vi "BioMapWriteCore.vi"(6 "conv. coeff.":sgl=655.0, 7 "Image in":dbl[][][](array[numeric]), 8 "error in":errorcluster, 9 "Y_img":i32, 10 "Image Params":T1={"File Header"={"Start Position"=[], "StepWidth"=[0.05, 0.05], "Dimension"=[], "SpecLength"=10000}, "mzCali."=[0.0, 1.0, 0.0], "m/z_Array"=[0.0, 1.0, 0.0], "SampleRate"=0.0, "TrigDelay"=0.0, "file refnum"=refnum, "file path"=path "", "PeakOI"=[], "Binning"={"Enable"=FALSE, "BinType"=enum."ByScreen", "BinWidth"=0.5, "Maximum"=0.0, "Minimum"=0.0}} {"SampleRate" items=["50MS/s"=50000000.0, "100MS/s"=100000000.0, "125MS/s"=125000000.0, "200MS/s"=200000000.0, "250MS/s"=250000000.0, "500MS/s"=500000000.0, "1GS/s"=1000000000.0, "1.6GS/s"=1600000000.0, "2GS/s"=2000000000.0, "4GS/s"=4000000000.0]}, 11 "data buffer in":refnum<queue>) -> (0 "error out":errorcluster, 2 "file refnum out":refnum<file>, 5 "Image out":dbl[][][](array[numeric]))   [LabVIEW 2014]
uses:
  BioMAPWriterCoreParams.ctl
  Files/BinaryHeader.ctl
  ControlDef/SampleRateSelector.ctl
  Binning/BinType.ctl
panel:
  out "#element":i32
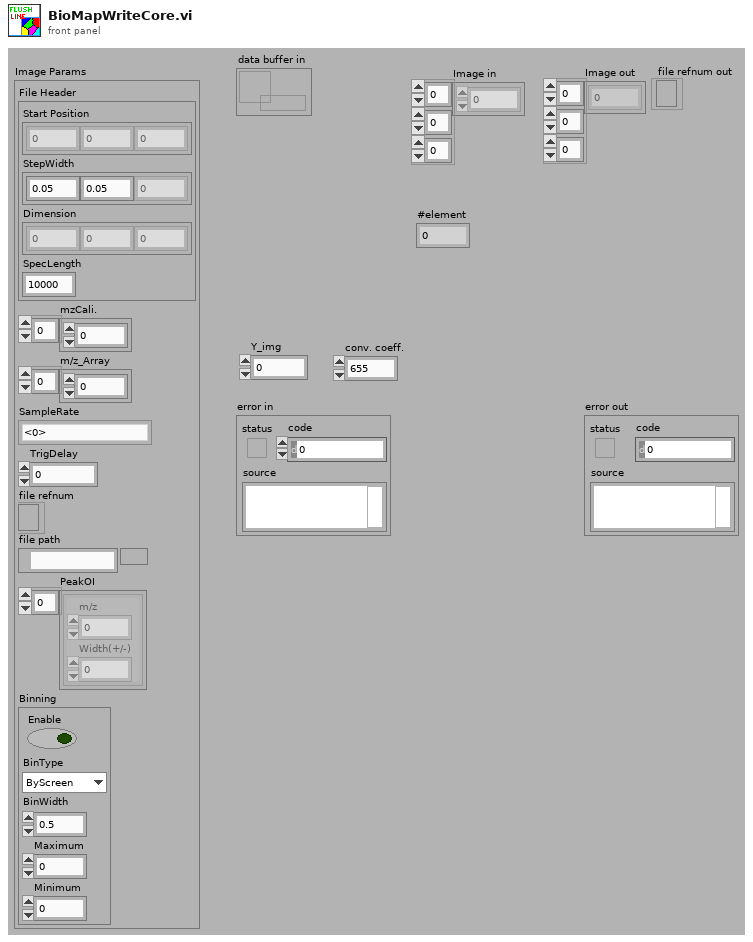
[diagram p1: front panel]
types:
  T1 = typedef "BioMAPWriterCoreParams.ctl" = cluster{"File Header":T2, "mzCali.":dbl[], "m/z_Array":dbl[], "SampleRate":T3, "TrigDelay":dbl, "file refnum":refnum<file>, "file path":path, "PeakOI":cluster{"m/z":dbl, "Width(+/-)":dbl}[], "Binning":cluster{"Enable":bool, "BinType":T4, "BinWidth":dbl, "Maximum":dbl, "Minimum":dbl}}
  T2 = typedef "BinaryHeader.ctl" = cluster{"Start Position":dbl[], "StepWidth":dbl[], "Dimension":i32[], "SpecLength":i32}
  T3 = typedef "SampleRateSelector.ctl" = dbl
  T4 = typedef "BinType.ctl" = enum16{"ByTime", "ByScreen", "ByMass", "ToUnitMass"}
  T5 = enum16{"big-endian, network order", "native, host order", "little-endian"}
  T6 = cluster{"Average":i32, "X (Img)":i32, "Y (Img)":i32, "Spectra":sgl[]}[]
  T7 = cluster{"Average":i32, "X (Img)":i32, "Y (Img)":i32, "Spectra":sgl[]}
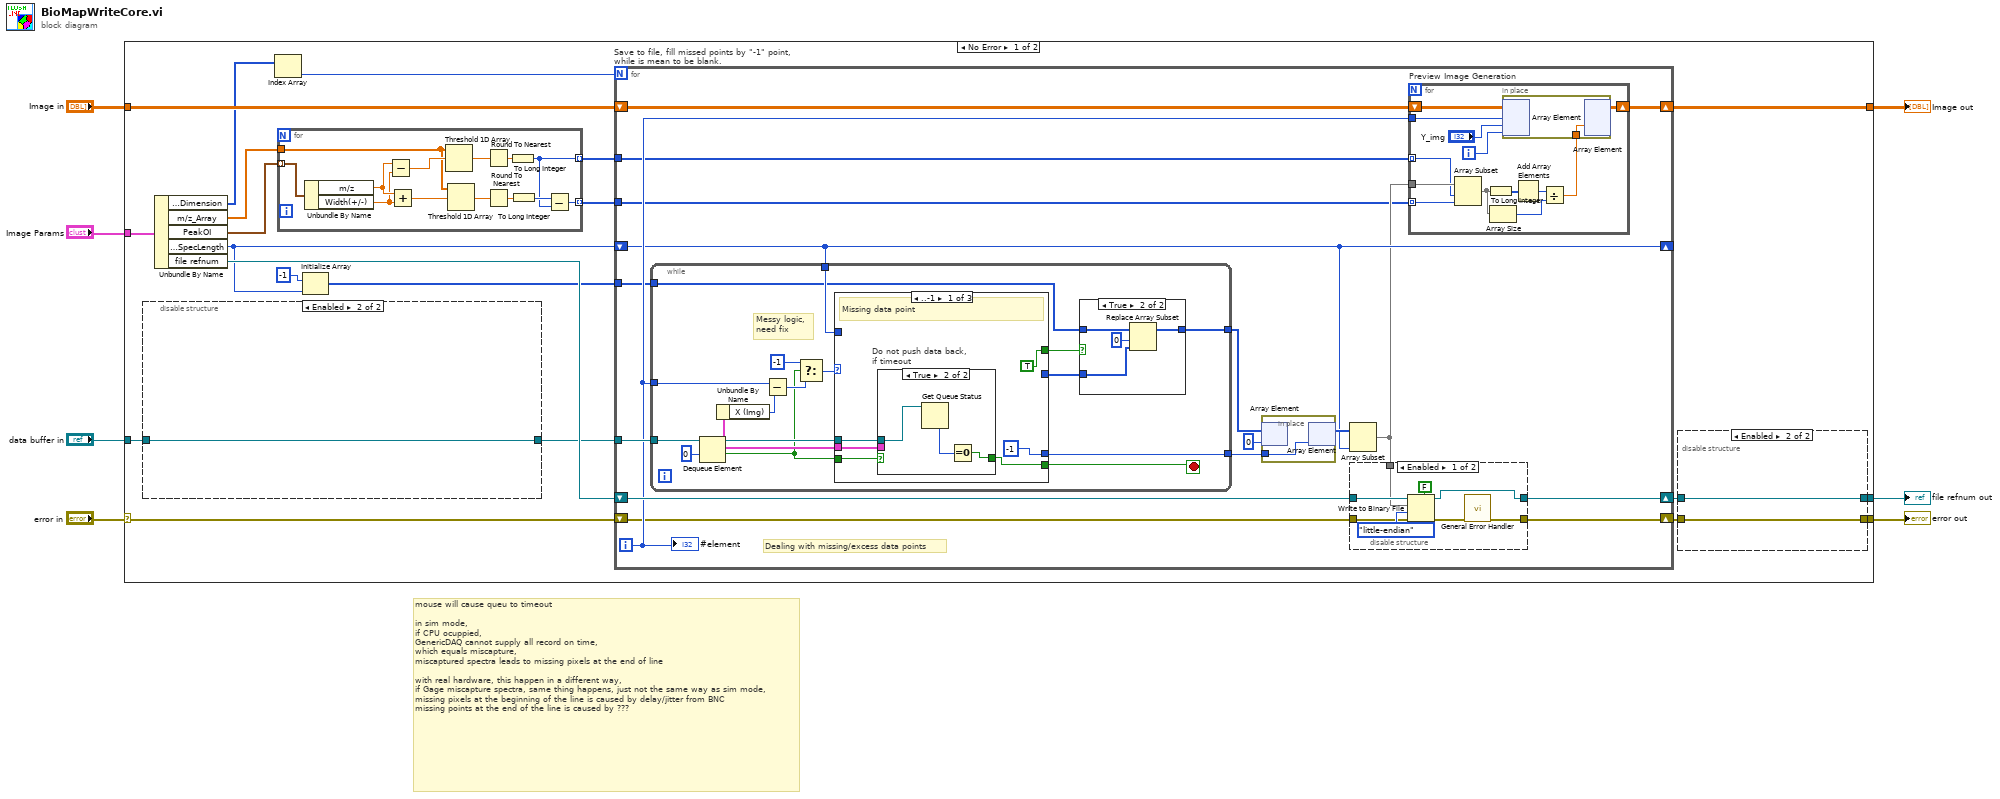
[diagram p0: block diagram]
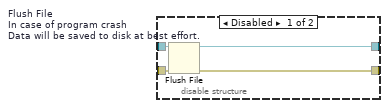
[diagram p2: hidden frame]
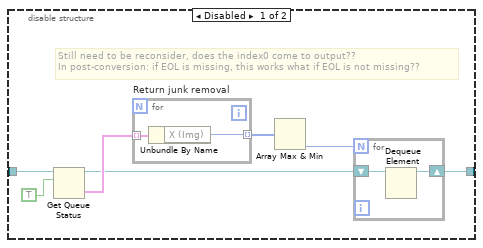
[diagram p3: hidden frame]
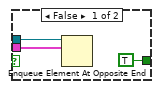
[diagram p6: hidden frame]
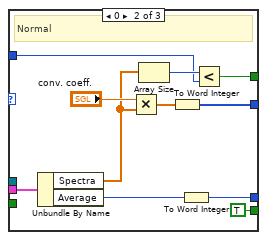
[diagram p7: hidden frame]
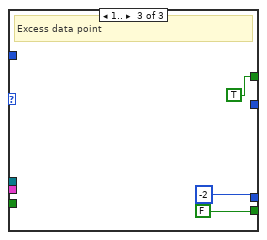
[diagram p8: hidden frame]
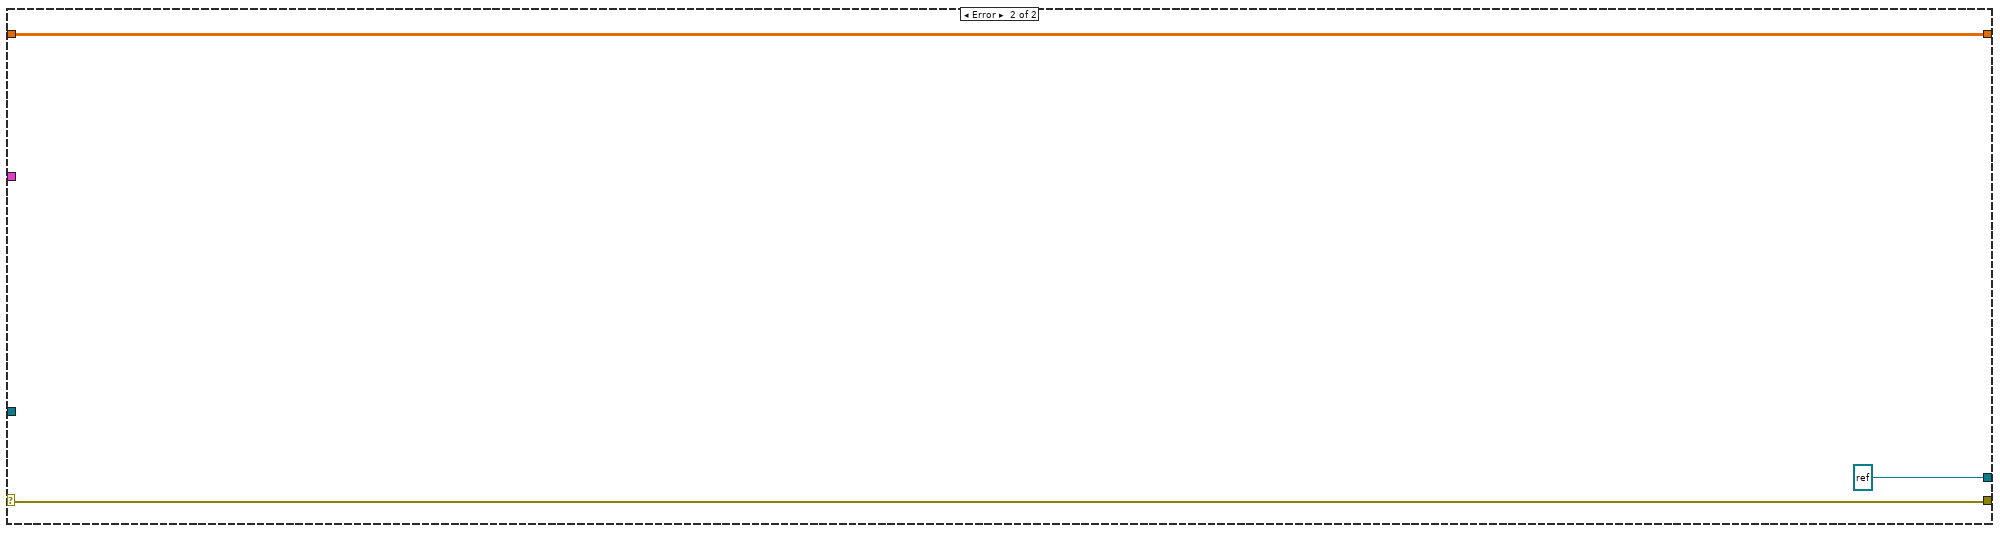
[diagram p9: hidden frame]
diagram:
  # "mouse will cause queu to timeout\n\nin sim mode, \nif CPU ocuppied,\nGenericDAQ cannot supply all record on time,\nwhich equals miscapture,\nmiscaptured spectra leads to missing pixels at the end of line\n\nwith real hardware, this happen in a different way,\nif Gage miscapture spectra, same thing happens, just not the same way as sim mode,\nmissing pixels at the beginning of the line is caused by delay/jitter from BNC\nmissing points at the end of the line is caused by ???"
  n1 = case shown="No Error" "error in" {
    selector: "error in" -> [w24 w150]
    tunnel: [w27 w148] -> w7
    tunnel: [w15 w150] -> w6
    tunnel: [w17 refnum<file> refnum ("file refnum")] -> w5
    tunnel: "Image in" -> [w25 w148]
    tunnel: "data buffer in" -> [w14 _]
    tunnel: "Image Params" -> [w12 _]
    frame No Error {
      n2 = disable-structure shown="Enabled" {
        disable-tunnel: w14 -> [w51 w58]
        disable-tunnel: [w49 w58] -> w20
        frame Disabled {
          # "Still need to be reconsider, does the index0 come to output??\nIn post-conversion: if EOL is missing, this works what if EOL is not missing??"
          # "Dealing with uncontroled laser. Data points from stage returning will be ignored."
          n3 = Get Queue Status(queue=w51, return elements? (F)=TRUE) -> (queue out=w50:refnum<queue>, elements=w53:T6)  [unwired: 1 in, 6 out]
          n4 = for "Return junk removal" {
            tunnel: w53 -> [w57] mode=indexing
            tunnel: [w56] -> w48 mode=indexing
            n5 = Unbundle By Name(w57) -> ("X (Img)"=w56:i32)
          }
          n6 = Array Max & Min(array=w48) -> (min index (indices)=w47:i32)  [unwired: 3 out]
          n7 = for {
            N: w47 -> [_]
            shift-right: [w54] -> w49
            shift-left: w50 -> [w55]
            n8 = Dequeue Element(queue=w55) -> (queue out=w54:refnum<queue>)  [unwired: 2 in, 3 out]
          }
        }
        frame Enabled {
          # "batch binning"
        }
      }
      n9 = Unbundle By Name(w12) -> ("File Header.Dimension"=w23:i32[], "m/z_Array"=w11:dbl[], "PeakOI"=w10:cluster{"m/z":dbl, "Width(+/-)":dbl}[], "File Header.SpecLength"=w13:i32, "file refnum"=w22:refnum<file>)
      n10 = Index Array(array=w23) -> (element=w21:i32)  [unwired: 1 in]
      n11 = for "Preview Image Generation" {
        tunnel: w10 -> [w46] mode=indexing
        tunnel: w11 -> [w42]
        tunnel: [w35] -> w9 mode=indexing
        tunnel: [w34] -> w8 mode=indexing
        n12 = Unbundle By Name(w46) -> ("m/z"=w45:dbl, "Width(+/-)"=w44:dbl)
        n13 = Subtract(x=w45, y=w44) -> (x-y=w43:dbl)
        n14 = Add(x=w45, y=w44) -> (x+y=w41:dbl)
        n15 = Threshold 1D Array(2:w43, 3:w42) -> (0:w40:dbl)  [unwired: 1 in]
        n16 = Threshold 1D Array(2:w41, 3:w42) -> (0:w39:dbl)  [unwired: 1 in]
        n17 = Round To Nearest(number=w40) -> (nearest integer value=w37:dbl)
        n18 = Round To Nearest(number=w39) -> (nearest integer value=w38:dbl)
        n19 = To Long Integer(number=w37) -> (32bit integer=w35:i32)
        n20 = To Long Integer(number=w38) -> (32bit integer=w36:i32)
        n21 = Subtract(x=w36, y=w35) -> (x-y=w34:i32)
      }
      n22 = Initialize Array(i16 -1 ("element"), w13) -> (w18:i16[])
      n23 = for "Save to file, fill missed points by \"-1\" point, while is mean to be blank." {
        N: w21 -> [_]
        shift-right: [w70] -> w16
        shift-left: w24 -> [w63]
        shift-right: [w72] -> w27
        shift-left: w25 -> [w71]
        tunnel: w20 -> [w75]
        shift-right: [w73] -> w26
        shift-left: w22 -> [w74]
        tunnel: w8 -> [w59]
        tunnel: w9 -> [w60]
        tunnel: w18 -> [w64]
        shift-right: [w62] -> _
        shift-left: w13 -> [w62]
        i -> [w65]
        # "Dealing with missing/excess data points"
        n24 = while {
          tunnel: w75 -> [w101]
          tunnel: [w95] -> w67
          tunnel: w62 -> [w94]
          tunnel: [w89] -> w66
          tunnel: w65 -> [w90]
          tunnel: w64 -> [w87]
          stop <- w93 stop-if-true
          # "Messy logic,\nneed fix"
          n25 = Dequeue Element(queue=w101, timeout in ms (-1)=0) -> (queue out=w97:refnum<queue>, element=w96:T7, timed out?=w86:bool)  [unwired: 1 in, 1 out]
          n26 = Unbundle By Name(w96) -> ("X (Img)"=w99:i32)
          n27 = Subtract(x=w90, y=w99) -> (x-y=w98:i32)
          n28 = Select(t=-1, s=w86, f=w98) -> (s? t:f=w92:i32)
          n29 = case shown="..-1" w92 {
            tunnel: w97 -> [w110 _ _]
            tunnel: w96 -> [w109 w129 _]
            tunnel: [i16 -1 ("Average") w127 i16 -2 ("Average")] -> w95
            tunnel: w94 -> [_ w122 _]
            tunnel: [w107 TRUE FALSE] -> w93
            tunnel: [_ w121 _] -> w88
            tunnel: [TRUE w120 TRUE] -> w85
            tunnel: w86 -> [w108 _ _]
            frame ..-1 {
              # "Missing data point"
              n30 = case "Do not push data back, \nif timeout" shown="True" w108 {
                tunnel: w110 -> [w115 w118]
                tunnel: w109 -> [w114 _]
                tunnel: [TRUE w116] -> w107
                frame False {
                  n31 = Enqueue Element At Opposite End(queue=w115, element=w114) -> ()  [unwired: 2 in, 3 out]
                }
                frame True {
                  n32 = Get Queue Status(queue=w118) -> (# elements in queue=w117:i32)  [unwired: 2 in, 7 out]
                  n33 = Equal To 0?(x=w117) -> (x = 0?=w116:bool)
                }
              }
            }
            frame 0 {
              # "Normal"
              n34 = Unbundle By Name(w129) -> ("Spectra"=w119:sgl[], "Average"=w126:i32)
              n35 = Multiply(x="conv. coeff.", y=w119) -> (x*y=w128:sgl[])
              n36 = Array Size(array=w119) -> (size(s)=w123:i32)
              n37 = To Word Integer(number=w128) -> (16bit integer=w121:i16[])
              n38 = To Word Integer(number=w126) -> (16bit integer=w127:i16)
              n39 = Less?(x=w123, y=w122) -> (x < y?=w120:bool)
            }
            frame 1.. {
              # "Excess data point"
            }
          }
          n40 = case shown="True" w85 {
            tunnel: [w102 w106] -> w89
            tunnel: w88 -> [w102 w104]
            tunnel: w87 -> [_ w105]
            frame False {
            }
            frame True {
              n41 = Replace Array Subset(array=w105, new element=w104, index=0) -> (w106:i16[])
            }
          }
        }
        n42 = in-place {
          in-place-border: w67 -> [w147]
          n43 = in-place-array #1(w66, 0) -> ()  [unwired: 1 out]
          n44 = in-place-array #1(w147) -> (w68:i16[])  [unwired: 1 out]
        }
        n45 = Array Subset(array=w68, length=w62) -> (w61:i16[])  [unwired: 1 in]
        n46 = disable-structure shown="Enabled" {
          disable-tunnel: w74 -> [w83 w84]
          disable-tunnel: [w82 w84] -> w73
          disable-tunnel: [w81 _] -> w70
          disable-tunnel: w63 -> [w77 _]
          disable-tunnel: w61 -> [w76 _]
          frame Enabled {
            n47 = Write to Binary File(file (use dialog)=w83, data=w76, error in=w77, 5:FALSE ("prepend array or string size? (T)"), 9:T5."little-endian" ("byte order (0:big-endian, network order)")) -> (refnum out=w82:refnum<file>, error out=w78:errorcluster)  [unwired: 1 in, 1 out]
            n48 = call <vilib>:"General Error Handler.vi"("error in (no error)"=w78) -> ("error out"=w81:errorcluster)  [unwired: 10 in, 4 out]
          }
          frame Disabled {
          }
        }
        n49 = for "Preview Image Generation" {
          shift-right: [w143] -> w72
          shift-left: w71 -> [w145]
          tunnel: w61 -> [w144]
          tunnel: w65 -> [w138]
          tunnel: w59 -> [w133] mode=indexing
          tunnel: w60 -> [w134] mode=indexing
          i -> [w137]
          n50 = Array Subset(array=w144, index=w134, length=w133) -> (w140:i16[])
          n51 = To Long Integer(number=w140) -> (32bit integer=w135:i32[])
          n52 = Array Size(array=w140) -> (size(s)=w141:i32)
          n53 = Add Array Elements(numeric array=w135) -> (sum=w142:i32)
          n54 = Divide(x=w142, y=w141) -> (x/y=w139:dbl)
          n55 = in-place {
            in-place-border: w139 -> [w146]
            n56 = in-place-array #2(w145, w138, "Y_img", w137) -> ()  [unwired: 1 out]
            n57 = in-place-array #2(w146) -> (w143:dbl[][][])  [unwired: 3 out]
          }
        }
        "#element" <- w65
      }
      n58 = disable-structure shown="Enabled" {
        disable-tunnel: w26 -> [w31 w33]
        disable-tunnel: [w30 w33] -> w17
        disable-tunnel: w16 -> [w29 w32]
        disable-tunnel: [w28 w32] -> w15
        frame Disabled {
          n59 = Flush File "Flush File\nIn case of program crash\nData will be saved to disk at best effort."(refnum=w31, error in=w29) -> (refnum out=w30:refnum<file>, error out=w28:errorcluster)
        }
        frame Enabled {
        }
      }
    }
    frame Error {
    }
  }
  "Image out" <- w7
  "error out" <- w6
  "file refnum out" <- w5
